vi "mediaIntesecaoBlue.vi"(11 "Array":T4[](array[typedef]) {"robots_blue"."height" format="%+4.3f"; "robots_blue"."pixel_y" format="%+4.3f"; "robots_blue"."pixel_x" format="%+4.3f"; "robots_blue"."orientation" format="%+4.3f"; "robots_blue"."y" format="%+4.3f"; "robots_blue"."confidence" format="%4.3f"; "robots_blue"."x" format="%+4.3f"; "robots_yellow"."height" format="%+4.3f"; "robots_yellow"."pixel_y" format="%+4.3f"; "robots_yellow"."pixel_x" format="%+4.3f"; "robots_yellow"."orientation" format="%+4.3f"; "robots_yellow"."y" format="%+4.3f"; "robots_yellow"."confidence" format="%4.3f"; "robots_yellow"."x" format="%+4.3f"}) -> (3 "Array 2":T1[](array[typedef]) {"height" format="%+4.3f"; "pixel_y" format="%+4.3f"; "pixel_x" format="%+4.3f"; "orientation" format="%+4.3f"; "y" format="%+4.3f"; "confidence" format="%4.3f"; "x" format="%+4.3f"})   [LabVIEW 2018]
uses:
  SSL Detection Frame.ctl
  SSL Detection Robot.ctl
  <vilib>/Analysis/Matrix/Datatypes/RealMatrix.ctl
  SSL Detection Ball.ctl
  <vilib>/Analysis/Matrix/NI_Matrix.lvlib
panel:
  in  "Field Size 2":T3
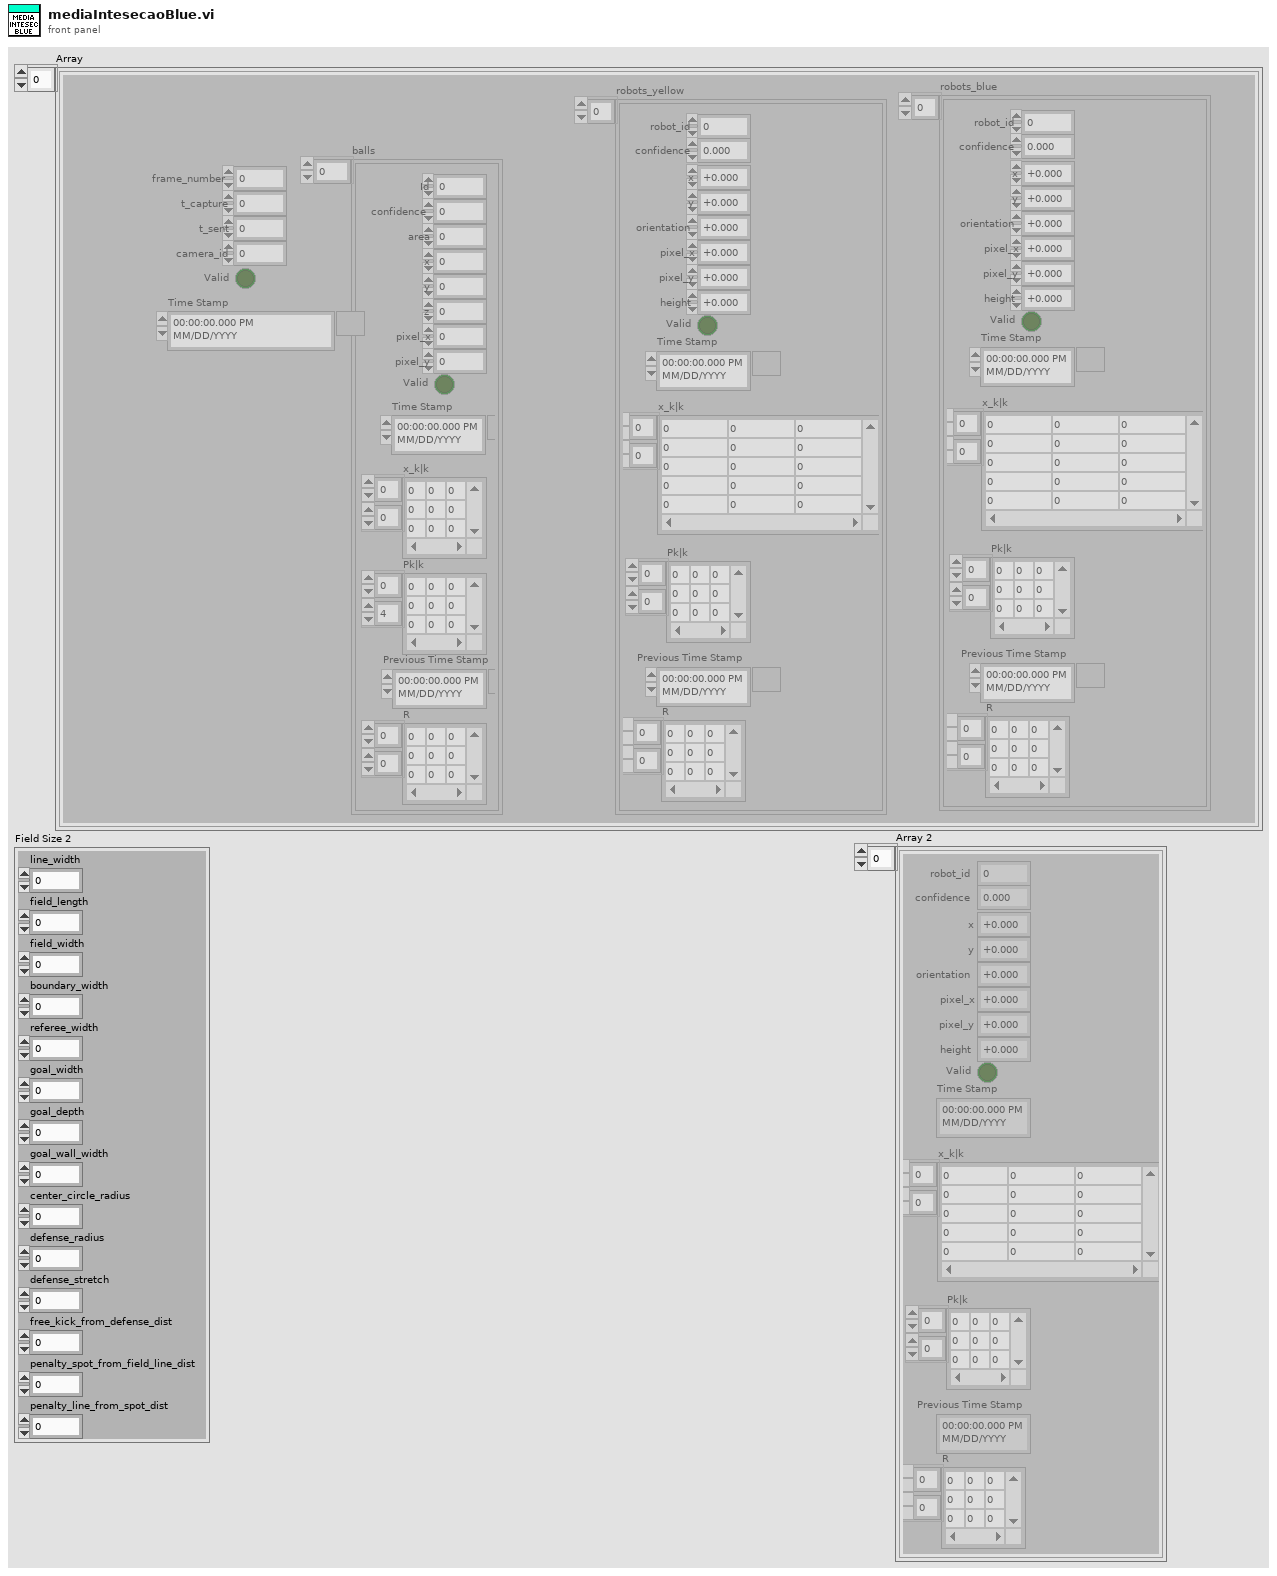
[diagram p1: front panel]
types:
  T1 = typedef "SSL Detection Robot.ctl" = cluster{"x":sgl, "robot_id":u32, "confidence":sgl, "y":sgl, "orientation":sgl, "pixel_x":sgl, "pixel_y":sgl, "height":sgl, "Valid":bool, "Time Stamp":timestamp, "x_k|k":T2, "Pk|k":T2, "Previous Time Stamp":timestamp, "R":T2}
  T2 = typedef "NI_Matrix.lvlib/RealMatrix.ctl" = dbl[][]
  T3 = cluster{"line_width":u32, "field_length":u32, "field_width":u32, "boundary_width":u32, "referee_width":u32, "goal_width":u32, "goal_depth":u32, "goal_wall_width":u32, "center_circle_radius":u32, "defense_radius":u32, "defense_stretch":u32, "free_kick_from_defense_dist":u32, "penalty_spot_from_field_line_dist":u32, "penalty_line_from_spot_dist":u32}
  T4 = typedef "SSL Detection Frame.ctl" = cluster{"frame_number":u32, "t_capture":dbl, "t_sent":dbl, "camera_id":u32, "robots_yellow":T1[], "robots_blue":T1[], "balls":T5[], "Valid":bool, "Time Stamp":timestamp}
  T5 = typedef "SSL Detection Ball.ctl" = cluster{"x":sgl, "area":u32, "confidence":sgl, "y":sgl, "z":sgl, "pixel_x":sgl, "pixel_y":sgl, "Valid":bool, "Time Stamp":timestamp, "x_k|k":T2, "Pk|k":T2, "Id":u32, "Previous Time Stamp":timestamp, "R":T2}
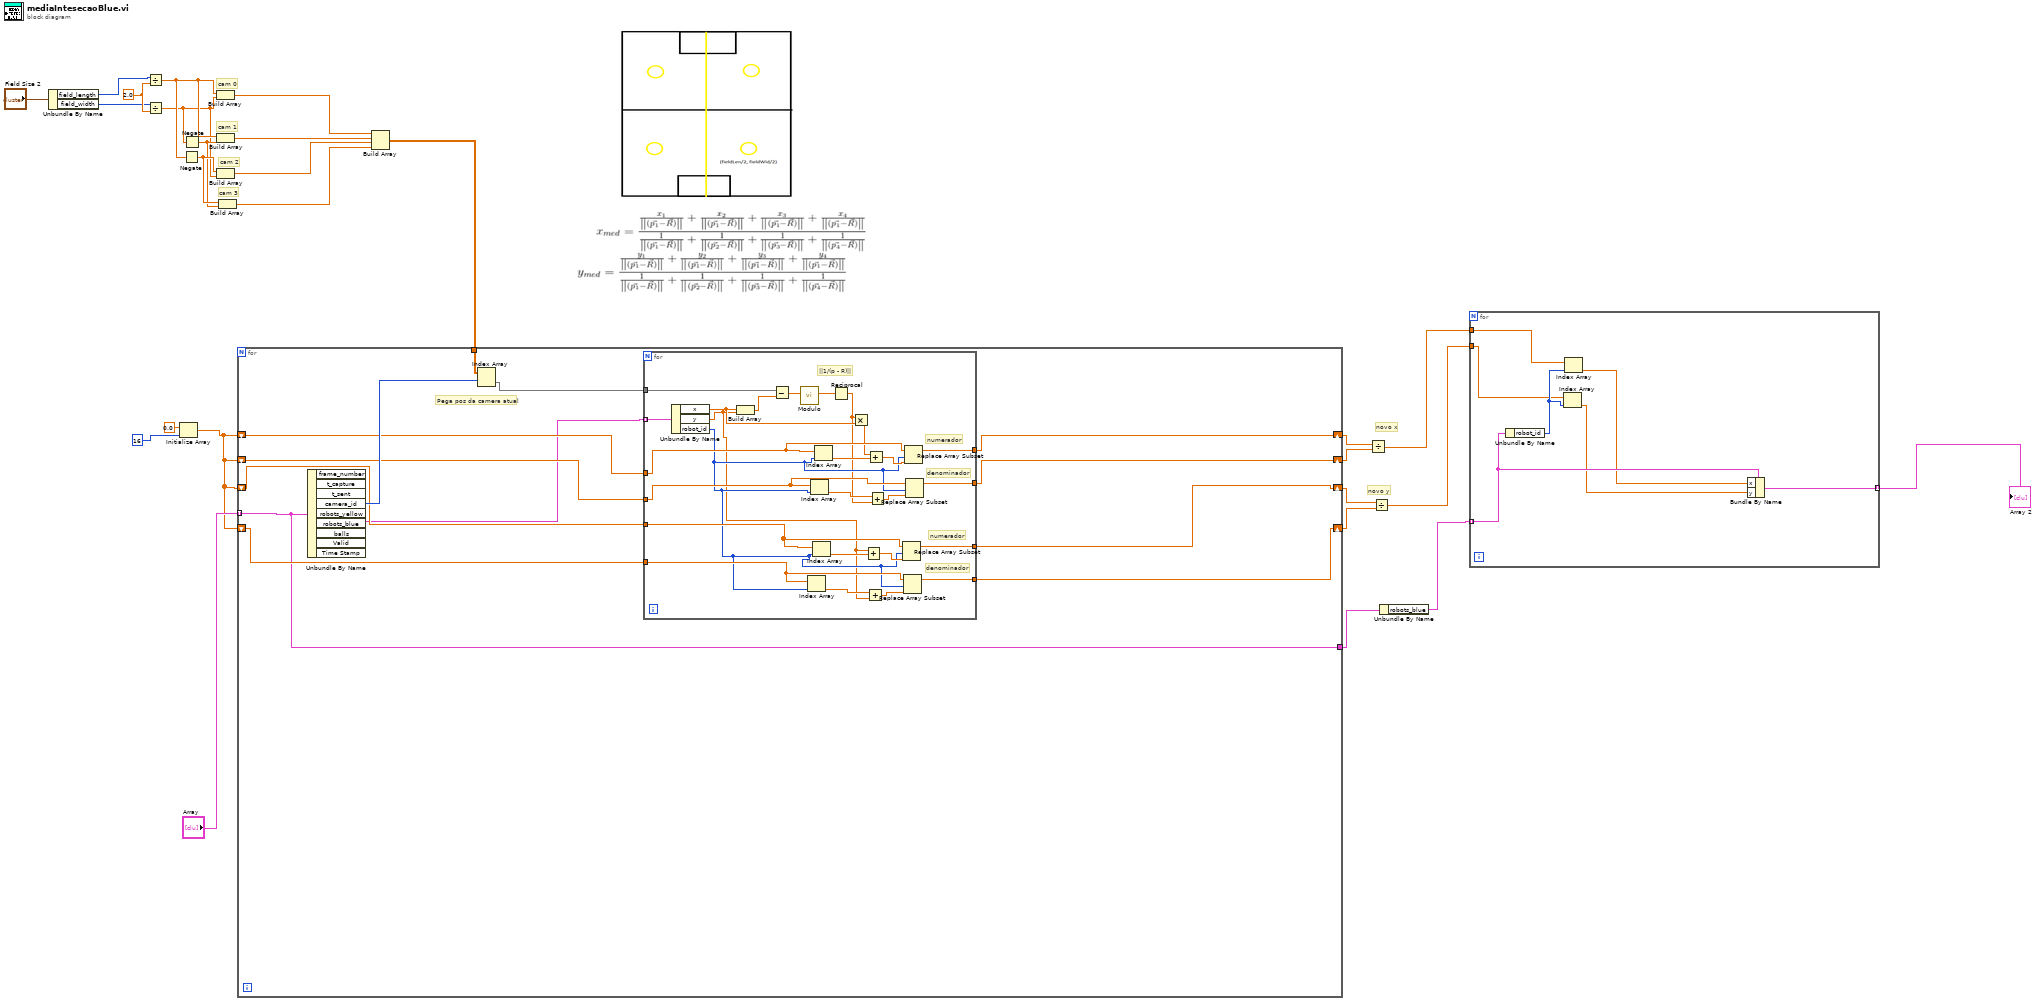
[diagram p0: block diagram]
diagram:
  w24 = 2.0 ("y")
  # "novo y"
  # "novo x"
  # "cam 3"
  # "cam 2"
  # "cam 1"
  # "cam 0"
  n1 = Unbundle By Name("Field Size 2") -> ("field_length"=w23:u32, "field_width"=w22:u32)
  n2 = Divide(x=w23, y=w24) -> (x/y=w20:dbl)
  n3 = Divide(x=w22, y=w24) -> (x/y=w18:dbl)
  n4 = Initialize Array(0.0 ("element"), 16 ("dimension size")) -> (w1:dbl[])
  n5 = Negate(x=w20) -> (-x=w21:dbl)
  n6 = Negate(x=w18) -> (-x=w19:dbl)
  n7 = Build Array(w20, w18) -> (w17:dbl[])
  n8 = Build Array(w20, w19) -> (w16:dbl[])
  n9 = Build Array(w21, w18) -> (w15:dbl[])
  n10 = Build Array(w21, w19) -> (w14:dbl[])
  n11 = Build Array(w17, w16, w15, w14) -> (w13:dbl[][])
  n12 = for {
    tunnel: "Array" -> [w28] mode=indexing
    tunnel: w13 -> [w39]
    shift-right: [w34] -> w10
    shift-left: w1 -> [w36]
    shift-right: [w33] -> w9
    shift-left: w1 -> [w35]
    shift-right: [w30] -> w8
    shift-left: w1 -> [w32]
    shift-right: [w29] -> w7
    shift-left: w1 -> [w31]
    tunnel: [w28] -> w3
    # "Pega pos da camera atual"
    n13 = Unbundle By Name(w28) -> ("camera_id"=w38:u32, "robots_blue"=w27:T1[])  [unwired: 7 out]
    n14 = Index Array(array=w39, index (row)=w38) -> (element=w37:dbl[])  [unwired: 1 in]
    n15 = for {
      tunnel: w27 -> [w65] mode=indexing
      tunnel: w37 -> [w63]
      tunnel: w36 -> [w57]
      tunnel: w35 -> [w53]
      tunnel: [w59] -> w34
      tunnel: [w58] -> w33
      tunnel: w32 -> [w46]
      tunnel: w31 -> [w45]
      tunnel: [w42] -> w30
      tunnel: [w41] -> w29
      # "denominador"
      # "numerador"
      # "denominador"
      # "numerador"
      # "||1/(p - R)||"
      n16 = Unbundle By Name(w65) -> ("x"=w60:sgl, "y"=w40:sgl, "robot_id"=w44:u32)
      n17 = Build Array(w60, w40) -> (w64:sgl[])
      n18 = Subtract(x=w63, y=w64) -> (x-y=w62:dbl[])
      n19 = call "Modulo.vi"("2D vector"=w62) -> ("Modulo"=w61:dbl)  [unwired: 10 in]
      n20 = Index Array(array=w45, index=w44) -> (element=w48:dbl)
      n21 = Index Array(array=w53, index=w44) -> (element=w52:dbl)
      n22 = Index Array(array=w46, index=w44) -> (element=w50:dbl)
      n23 = Index Array(array=w57, index=w44) -> (element=w55:dbl)
      n24 = Reciprocal(x=w61) -> (1/x=w43:dbl)
      n25 = Multiply(x=w43, y=w60) -> (x*y=w56:dbl)
      n26 = Add(x=w40, y=w50) -> (x+y=w49:dbl)
      n27 = Add(x=w48, y=w40) -> (x+y=w47:dbl)
      n28 = Add(x=w56, y=w55) -> (x+y=w54:dbl)
      n29 = Add(x=w52, y=w43) -> (x+y=w51:dbl)
      n30 = Replace Array Subset(array=w46, new element=w49, index=w44) -> (w42:dbl[])
      n31 = Replace Array Subset(array=w45, new element=w47, index=w44) -> (w41:dbl[])
      n32 = Replace Array Subset(array=w57, new element=w54, index=w44) -> (w59:dbl[])
      n33 = Replace Array Subset(array=w53, new element=w51, index=w44) -> (w58:dbl[])
    }
  }
  n34 = Divide(x=w10, y=w9) -> (x/y=w6:dbl[])
  n35 = Divide(x=w8, y=w7) -> (x/y=w5:dbl[])
  n36 = Unbundle By Name(w3) -> ("robots_blue"=w2:T1[])
  n37 = for {
    tunnel: w6 -> [w71]
    tunnel: w5 -> [w69]
    tunnel: w2 -> [w72] mode=indexing
    tunnel: [w66] -> w4 mode=indexing
    n38 = Unbundle By Name(w72) -> ("robot_id"=w70:u32)
    n39 = Index Array(array=w69, index=w70) -> (element=w67:dbl)
    n40 = Index Array(array=w71, index=w70) -> (element=w68:dbl)
    n41 = Bundle By Name(cluster=w72, "x"=w68, "y"=w67) -> (w66:T1)
  }
  "Array 2" <- w4
